vi "JSON Unescape.vi"(1 "Escaped JSON String":string) -> (0 "JSON String":string)   [LabVIEW 2013, in "LV JSON.lvlib"]
uses:
  LV JSON.lvlib
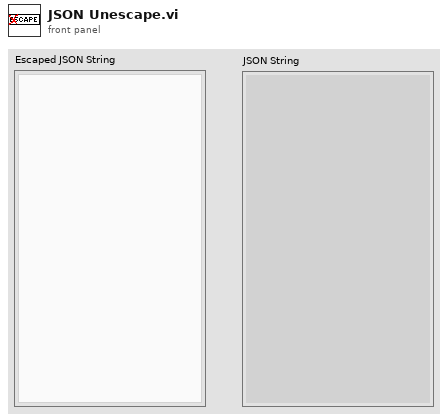
[diagram p1: front panel]
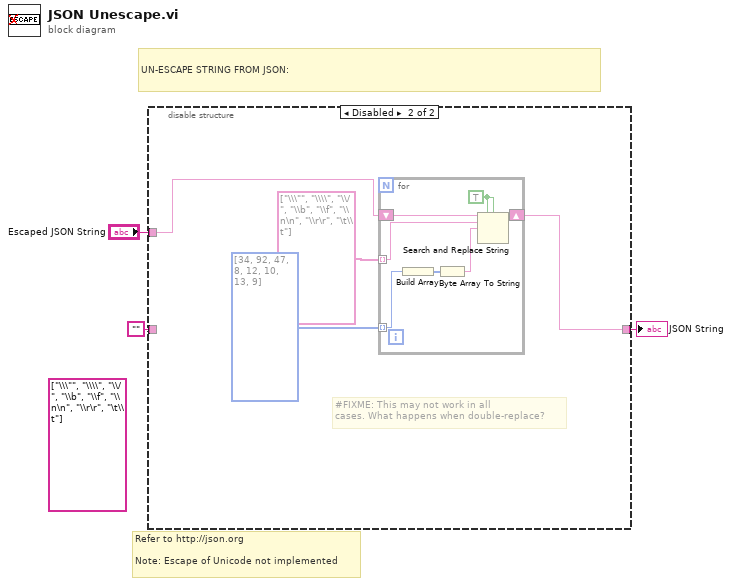
[diagram p0: block diagram]
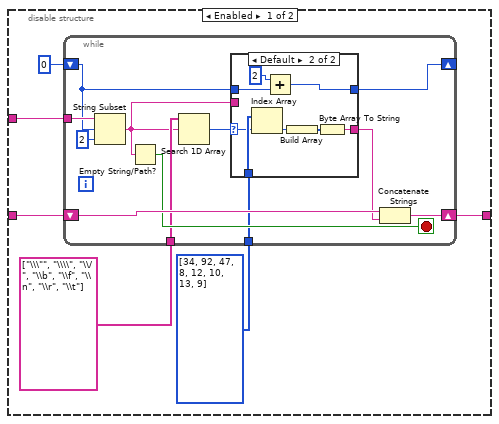
[diagram p2: hidden frame]
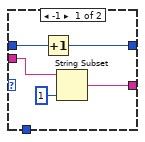
[diagram p3: hidden frame]
diagram:
  (unwired) string[] ["\\\"", "\\\\", "\\/", "\\b", "\\f", "\\n\n", "\\r\r", "\t\\t"] ("Array 2")
  # "UN-ESCAPE STRING FROM JSON:"
  # "Refer to http://json.org\n\nNote: Escape of Unicode not implemented"
  n1 = disable-structure shown="Disabled" {
    disable-tunnel: "" -> [w9 _]
    disable-tunnel: "Escaped JSON String" -> [w8 w36]
    disable-tunnel: [w7 w35] -> w2
    frame Enabled {
      n2 = while {
        shift-right: [w20] -> w7
        shift-left: w9 -> [w21]
        shift-right: [w13] -> _
        shift-left: 0 ("length (rest)") -> [w14]
        tunnel: w8 -> [w18]
        tunnel: string[] ["\\\"", "\\\\", "\\/", "\\b", "\\f", "\\n", "\\r", "\\t"] ("Array 2") -> [w16]
        tunnel: u8[] [34, 92, 47, 8, 12, 10, 13, 9] ("unsigned byte array") -> [w12]
        stop <- w19 stop-if-true
        n3 = String Subset(string=w18, offset (0)=w14, length (rest)=2 ("length (rest)")) -> (substring=w11:string)
        n4 = Empty String/Path?(string/path=w11) -> (empty?=w19:bool)
        n5 = Search 1D Array(1D array=w16, element=w11) -> (index of element=w15:i32)  [unwired: 1 in]
        n6 = case shown="Default" w15 {
          selector: w15 -> [_ w28]
          tunnel: w14 -> [w26 w34]
          tunnel: [w25 w32] -> w13
          tunnel: w12 -> [_ w29]
          tunnel: w11 -> [w23 _]
          tunnel: [w22 w27] -> w10
          frame -1 {
            n7 = Increment(x=w26) -> (x+1=w25:i32)
            n8 = String Subset(string=w23, length (rest)=1 ("length (rest)")) -> (substring=w22:string)  [unwired: 1 in]
          }
          frame Default {
            n9 = Index Array(array=w29, index=w28) -> (element=w30:u8)
            n10 = Add(x=2 ("y"), y=w34) -> (x+y=w32:i32)
            n11 = Build Array(w30) -> (w31:u8[])
            n12 = Byte Array To String(unsigned byte array=w31) -> (string=w27:string)
          }
        }
        n13 = Concatenate Strings(w21, w10) -> (w20:string)
      }
    }
    frame Disabled {
      # "#FIXME: This may not work in all\ncases. What happens when double-replace?"
      n14 = for {
        tunnel: string[] ["\\\"", "\\\\", "\\/", "\\b", "\\f", "\\n\n", "\\r\r", "\t\\t"] ("Array 2") -> [w42] mode=indexing
        tunnel: u8[] [34, 92, 47, 8, 12, 10, 13, 9] ("unsigned byte array") -> [w40] mode=indexing
        shift-right: [w44] -> w35
        shift-left: w36 -> [w45]
        w43 = TRUE ("replace all? (F)")
        n15 = Build Array(w40) -> (w39:u8[])
        n16 = Byte Array To String(unsigned byte array=w39) -> (string=w41:string)
        n17 = Search and Replace String(replace all?=w43, case sensitive?=w43, input string=w45, search string=w42, replace string=w41) -> (result string=w44:string)  [unwired: 3 in, 3 out]
      }
    }
  }
  "JSON String" <- w2
